vi "CsTool-FreeSystemFill.vi"(1 "Handle Cluster":T1) -> (0 "Error Code":i32)   [LabVIEW 2022 SP3]
doc: "This VI frees the CompuScope system identified by Handle Cluster, which should have been obtained by using CsTool-GetSystem.vi. \n\nIf the call is successful, a 1 is returned in the Error Code indicator. Otherwise, an error code is returned. A descriptive error string may be obtained by using CsTool-ErrorHandler.vi.\n\nUntil CsTool-FreeSystem.vi is called, a system that was obtained by CsTool-GetSystem.vi, will be considered to be in use by the driver and will be unavailable for other processes.\n\nIf the user exits a LabVIEW CompuScope VI without freeing a CompuScope system handle, the system will remain inaccessible to other applications. The system can be manually freed using the driver's CompuScope Manager utility."
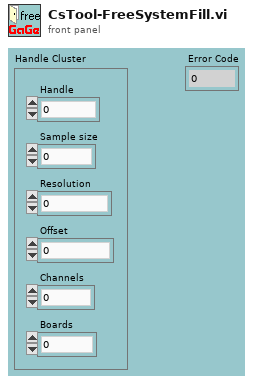
[diagram p1: front panel]
types:
  T1 = cluster{"Handle":u32, "Sample size":u32, "Resolution":i32, "Offset":i32, "Channels":u32, "Boards":u32}
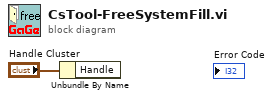
[diagram p0: block diagram]
diagram:
  n1 = Unbundle By Name("Handle Cluster") -> ()  [unwired: 1 out]
